vi "Set Dependency.vi"(8 "error in (no error)":errorcluster, 10 "Dependency":T1, 11 "DAQ_Engine in":refnum<class "DAQ_Engine.lvclass">) -> (0 "error out":errorcluster, 3 "DAQ_Engine out":refnum<class "DAQ_Engine.lvclass">)   [LabVIEW 2019, in "DAQ_Engine.lvclass"]
doc: "Developed by Kevin Thompson\nkevin@thompsonengineering.net\n\nCopyright 2018\nThompson Engineering, LLC"
uses:
  DAQ_Engine.lvclass
  DataTypes/Dependency--cluster.ctl
  Config/Config.lvclass
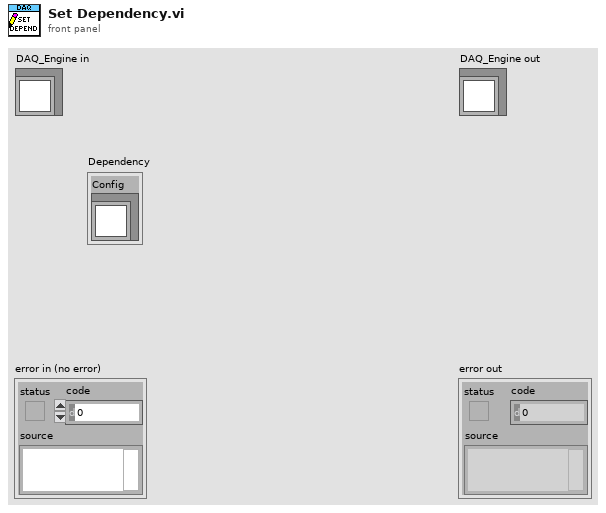
[diagram p1: front panel]
types:
  T1 = typedef "DAQ_Engine.lvclass/Dependency--cluster.ctl" = cluster{"Config":refnum<class "Config.lvclass">}
  T2 = typedef "DAQ_Engine.lvclass/ObjData--cluster.ctl" = cluster{"Settings":T3, "Public Events":T8, "Dependency":T1, "ReadData-placeholder":T9, "VISA-placeholder":refnum<visa-resource-name>, "MeasSettings":T4, "InverterDataAcqMode":T7, "RawDaqDataQ":T10, "Private Events":T11, "DAQState Data":T12}
  T3 = typedef "DAQ_Engine.lvclass/Settings--cluster.ctl" = cluster{"Simulation":bool, "Initial ErrReporting setting":i32, "Initial Measurement settings":T4, "BoardNum":T6, "Acquisition mode":T7, "DemoMode":bool}
  T4 = typedef "Measurement Config--cluster.ctl" = cluster{"Data Rate 9775":T5, "Data Rate 9215":u32, "Samples RMS 9215":u32, "Samples RMS 9775":u32}
  T5 = typedef "nicrio_cRIO-9775_ContinuousDataRates4ChansRing.ctl" = u16
  T6 = typedef "DAQ_Engine.lvclass/BoardNum--cluster.ctl" = cluster{"P1Sgl":u32, "P2":u32, "P3":u32}
  T7 = typedef "Acquisition Mode--cluster.ctl" = enum16{"3phase", "Single"}
  T8 = typedef "DAQ_Engine.lvclass/Public Events--cluster.ctl" = cluster{"DAQ_Engine.AsyncCmd Event":refnum<user-event>, "DAQ_Engine.AsyncMsg Event":refnum<user-event>, "stop process":refnum<user-event>, "DAQ_Engine.DAQStateChg Ev":refnum<user-event>, "DAQ_Engine.MeasSettingsChg Ev":refnum<user-event>, "DAQ_Engine.AcqModeChg Ev":refnum<user-event>}
  T9 = typedef "DAQ_Engine.lvclass/Read Data--cluster.ctl" = cluster{"Data":dbl}
  T10 = typedef "RawDAQDataQRef--cluster.ctl" = refnum<queue>
  T11 = typedef "DAQ_Engine.lvclass/Private Events--cluster.ctl" = cluster{"PrivateAsync Ev":refnum<user-event>}
  T12 = typedef "DAQ_Engine.lvclass/DAQStateEvData--cluster.ctl" = cluster{"DAQState":T13, "vData":variant}
  T13 = typedef "DAQState--enum.ctl" = enum16{"Unknown", "Stopped", "Running", "Error"}
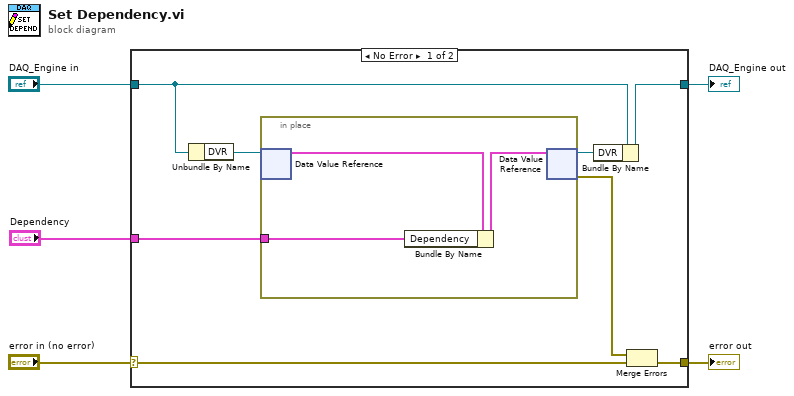
[diagram p0: block diagram]
diagram:
  n1 = case shown="No Error" "error in (no error)" {
    selector: "error in (no error)" -> [w7 w17]
    tunnel: [w8 w17] -> w4
    tunnel: [w9 w18] -> w2
    tunnel: "DAQ_Engine in" -> [w10 w18]
    tunnel: "Dependency" -> [w6 _]
    frame No Error {
      n2 = Unbundle By Name(w10) -> ("DVR"=w13:refnum<data-value>)
      n3 = in-place {
        in-place-border: w6 -> [w14]
        n4 = in-place-dvr #1(w13) -> (w16:T2)  [unwired: 1 out]
        n5 = Bundle By Name(cluster=w16, "Dependency"=w14) -> (w15:T2)
        n6 = in-place-dvr #1(w15) -> (w12:refnum<data-value>, w11:errorcluster)
      }
      n7 = Bundle By Name(cluster=w10, "DVR"=w12) -> (w9:refnum<class "DAQ_Engine.lvclass">)
      n8 = Merge Errors(w11, w7) -> (w8:errorcluster)
    }
    frame Error {
    }
  }
  "error out" <- w4
  "DAQ_Engine out" <- w2
